vi "GetLogfileNameByTime.vi"(8 "error in (no error)":errorcluster, 11 "FileExtension":string) -> (0 "error out":errorcluster, 3 "Name by Time":string)   [LabVIEW 2016, in "Log4Lv.lvlib"]
doc: "Use this template to build a VI to use as a subVI."
uses:
  Log4Lv.lvlib
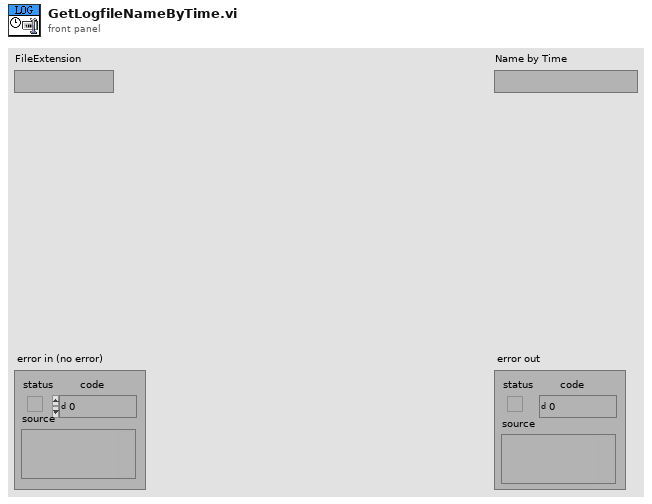
[diagram p1: front panel]
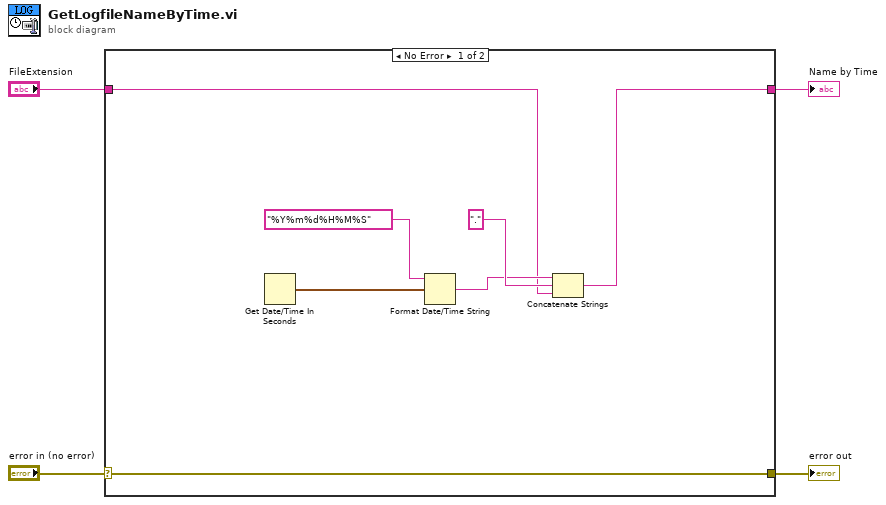
[diagram p0: block diagram]
diagram:
  n1 = case shown="No Error" "error in (no error)" {
    selector: "error in (no error)" -> [w9 w12]
    tunnel: [w9 w12] -> w3
    tunnel: [w6 _] -> w2
    tunnel: "FileExtension" -> [w5 _]
    frame No Error {
      n2 = Get Date/Time In Seconds() -> (seconds since 1Jan1904=w10:timestamp)
      n3 = Format Date/Time String(time format string (%c)="%Y%m%d%H%M%S", seconds (now)=w10) -> (date/time string=w7:string)  [unwired: 1 in]
      n4 = Concatenate Strings(w7, "." ("string"), w5) -> (w6:string)
    }
    frame Error {
    }
  }
  "error out" <- w3
  "Name by Time" <- w2
